vi "Get Server Loop.vi"(8 "error in (no error)":errorcluster, 11 "Websocket Server in":refnum<class "Websocket Server.lvclass">) -> (0 "error out":errorcluster, 2 "Server Loop":bool, 3 "Websocket Server out":refnum<class "Websocket Server.lvclass">)   [LabVIEW 2020, in "Stream-Websocket.lvlib" / "Websocket Server.lvclass"]
uses:
  Websocket Server.lvclass
  Websocket Server.lvclass/Websocket Server.ctl
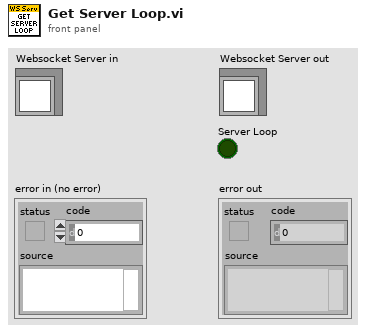
[diagram p1: front panel]
types:
  T1 = typedef "Stream-Websocket.lvlib/Websocket Server.lvclass/Ref Data.ctl" = cluster{"Listener":refnum<k5>, "Clients":refnum<class "Websocket Client.lvclass">[], "Server Loop":bool}
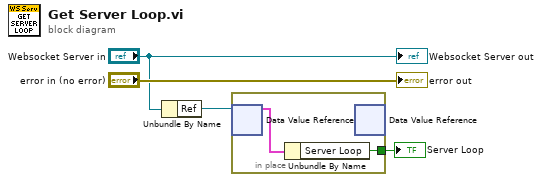
[diagram p0: block diagram]
diagram:
  n1 = Unbundle By Name("Websocket Server in") -> ("Ref"=w3:refnum<data-value>)
  n2 = in-place {
    in-place-border: [w5] -> w1
    n3 = in-place-dvr #1(w3) -> (w6:T1)  [unwired: 1 out]
    n4 = Unbundle By Name(w6) -> ("Server Loop"=w5:bool)
    n5 = in-place-dvr #1() -> ()  [unwired: 1 in, 2 out]
  }
  "Server Loop" <- w1
  "error out" <- "error in (no error)"
  "Websocket Server out" <- "Websocket Server in"
